vi "MEASURE_2dmapping.vi"() -> ()   [LabVIEW 2021]
uses:
  <vilib>/DAQmx/read.llb/DAQmx Read.vi
  <vilib>/DAQmx/read.llb/DAQmx Read (Counter U32 1Chan 1Samp).vi
  <vilib>/Analysis/baseanly.llb/Mean (DBL).vi
  <vilib>/DAQmx/create/channels.llb/DAQmx Create Channel (CI-Count Edges).vi
  <instrlib>/Keithley 24XX/Public/Data/Read (Multiple Points).vi
  <vilib>/DAQmx/miscellaneous.llb/DAQmx Fill In Error Info.vi
  <vilib>/Utility/file.llb/Write To Spreadsheet File (DBL).vi
  <instrlib>/Stanford Research 830/Stanford Research 830.lvlib
  <instrlib>/Keithley 2450/Keithley 2450.lvlib
  <resource>/objmgr/daqmx.rc
  <instrlib>/Keithley 24XX/Keithley 24XX.lvlib
  <vilib>/Analysis/NI_AALBase.lvlib
panel:
  out "XY Graph 4":cluster{dbl[], dbl[]}(graph)
  out "XY Graph 3":cluster{dbl[], dbl[]}(graph)
  out "top gate leaking":dbl
  out "top gate voltage":dbl format="%#_13g"
  in  "Compliance  Level (1uA)":dbl=1e-06
  in  "Source Mode  (0: Voltage)":u16(ring) items=["Voltage", "Current"]
  in  "Serial Configuration":T1={"Baud Rate"=9600, "Parity"=0, "Data Bits"=8, "Stop Bits"=10, "Flow Control"=0} {"Flow Control" items=["None", "XON/XOFF", "RTS/CTS", "XON/XOFF & RTS/CTS", "DTR/DSR", "XON/XOFF & DTR/DSR"]; "Stop Bits" items=["1.0"=10, "1.5"=15, "2.0"=20]; "Data Bits" items=["7"=7, "8"=8]; "Parity" items=["None", "Odd", "Even", "Mark", "Space"]; "Baud Rate" items=["300"=300, "600"=600, "1200"=1200, "2400"=2400, "4800"=4800, "9600"=9600, "19200"=19200]}
  in  "top gate address":refnum<visa-resource-name>="GPIB0::24::INSTR"
  in  "top gate thickness":dbl
  in  "bottom gate thickness":dbl
  in  "pure field (T)/pure doping (F)":bool
  in  "Clear Plot 2":bool
  out "XY Graph 2":cluster{dbl[], dbl[]}(graph)
  in  "accumulation":i32=100
  out "Waveform Chart 3":dbl[](graph)
  out "Numeric":dbl
  in  "Counter Channel":tag="/Dev1/PFI0"
  in  "error in":errorcluster
  out "loop run":i32
  in  "loop #":i32
  in  "Save data or not":bool=TRUE
  in  "path (folder + filename)":string="D:\\Kedar\\MoS2\\jw7_DJ_bulk_111213\\VvsHtr\\VvsHtr_300K"
  in  "Clear Plot":bool
  out "LOCKIN Measurement":dbl
  in  "Parameter (1: X)":u16(ring)=1 items=["X"=1, "Y"=2, "R"=3, "Theta"=4, "Channel 1"=5, "Channel 2"=6, "Aux In 1"=7, "Aux In 2"=8, "Aux In 3"=9, "Aux In 4"=10]
  out "back gate voltage":dbl format="%#_13g"
  out "back gate leaking":string="defbuffer1"
  in  "GATE STEP(mv)":i32
  in  "GATE Low Value (default 0)":dbl=1.0
  in  "GATE High Value":dbl=1.0
  in  "Function (0: Volts) 2":u16(ring) items=["Volts", "Current", "Resistance"]
  in  "Source Compaliance":dbl=1e-06
  in  "topgate address":refnum<visa-resource-name>="GPIB0::24::INSTR"
  in  "SD stabilization(S) 2":dbl format="%#_13g"
  in  "Sine Output Amplitude (1 V) 2":dbl=1.0
  in  "GATE / SD stablization 3":dbl format="%#_13g"
  in  "frequency":dbl format="%#_13g"
  in  "Input Connection (0: Single-Ended Voltage)":u16(ring) items=["Single-Ended Voltage", "Differential Voltage", "1 MOhm Current Gain", "100 MOhm Current Gain"]
  in  "LOCKIN address":refnum<visa-resource-name>="GPIB0::24::INSTR"
  # "Gate2450(back) Setting"
  # "Lock-in"
  # "Gate2401(top) Setting"
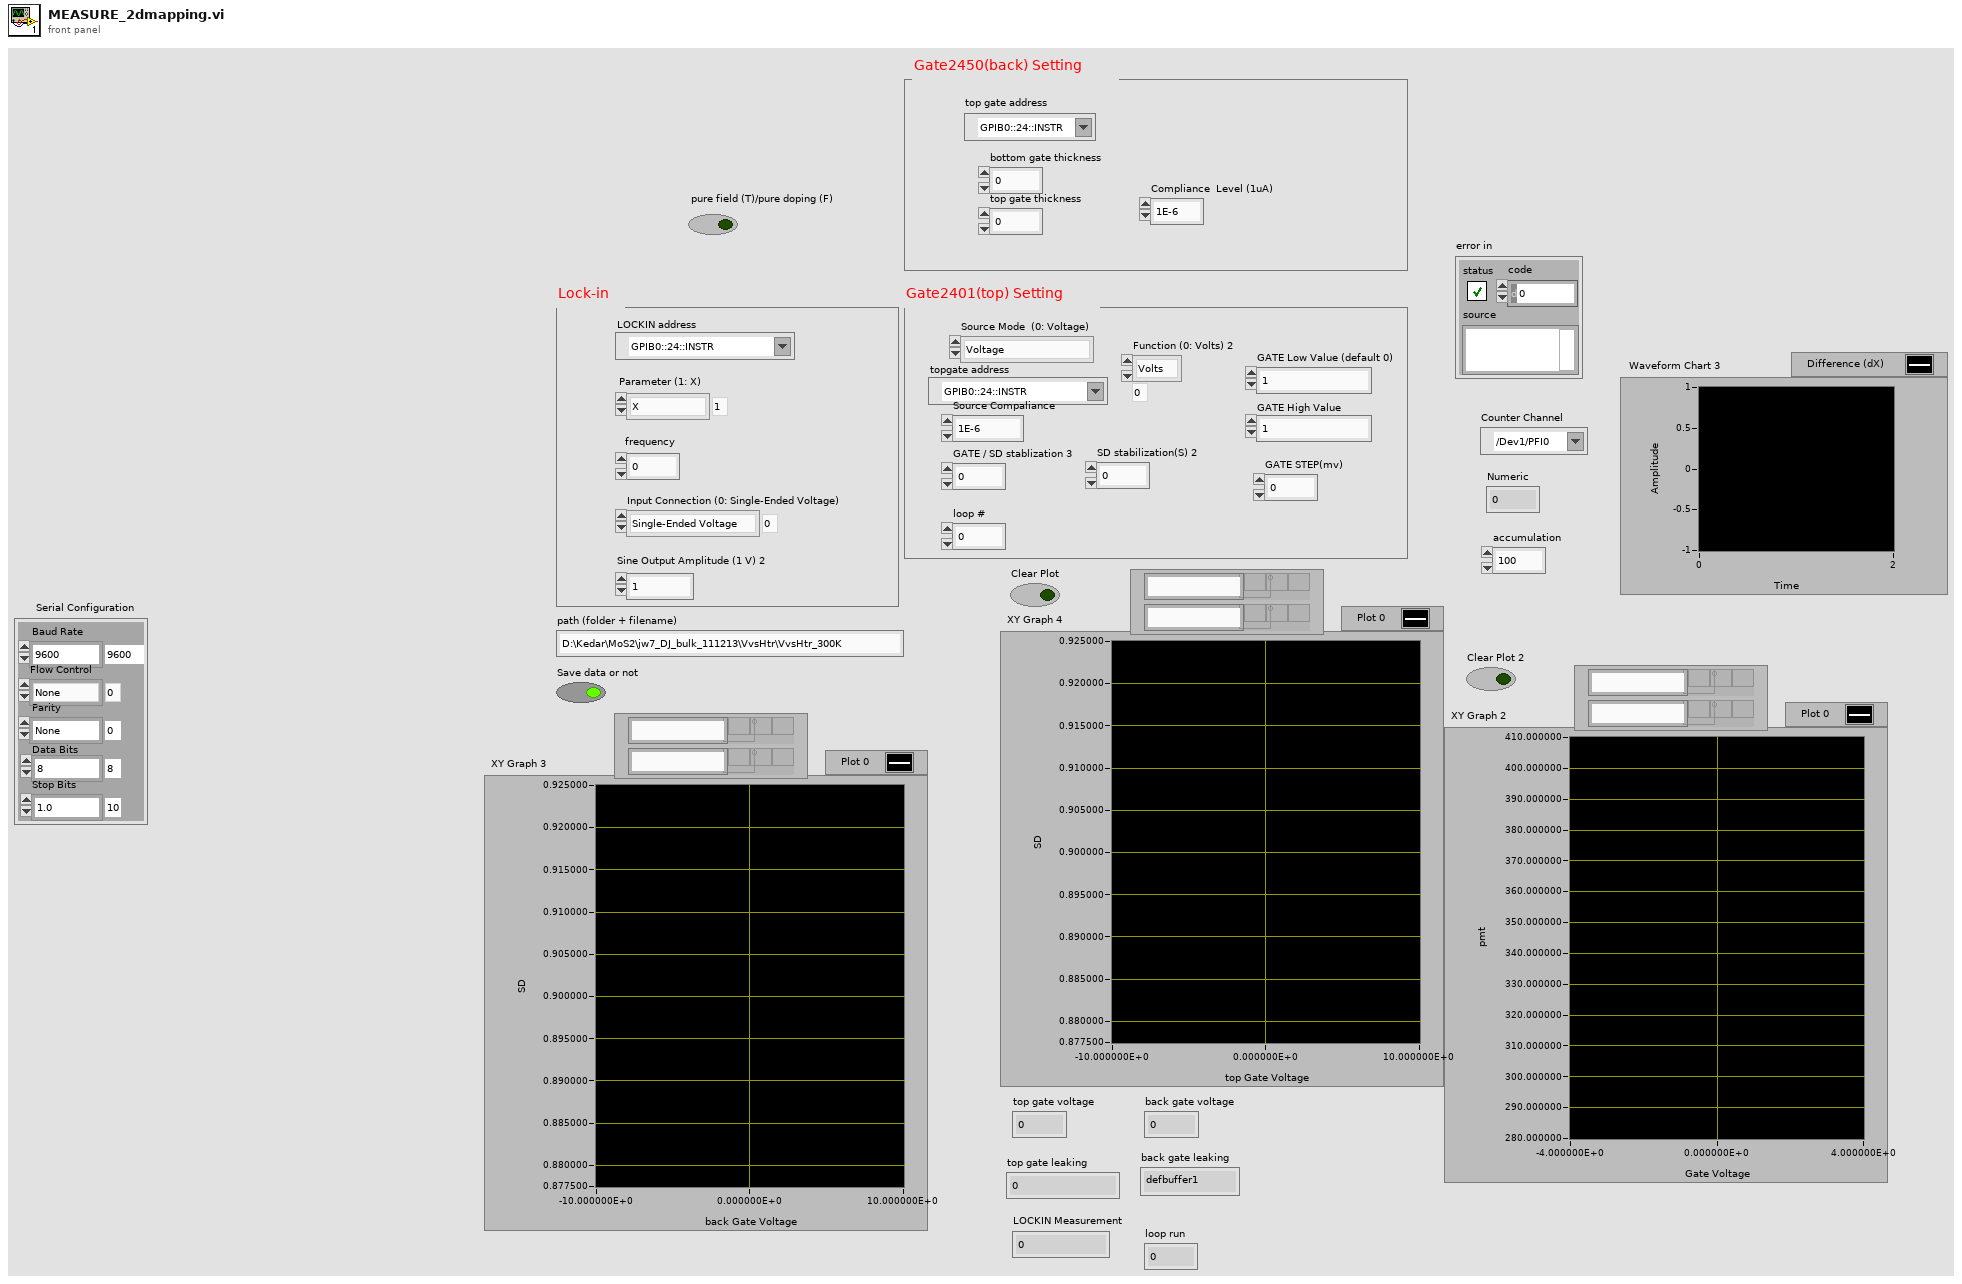
[diagram p1: front panel]
types:
  T1 = cluster{"Baud Rate":u32, "Parity":u16, "Data Bits":u16, "Stop Bits":u16, "Flow Control":u16}
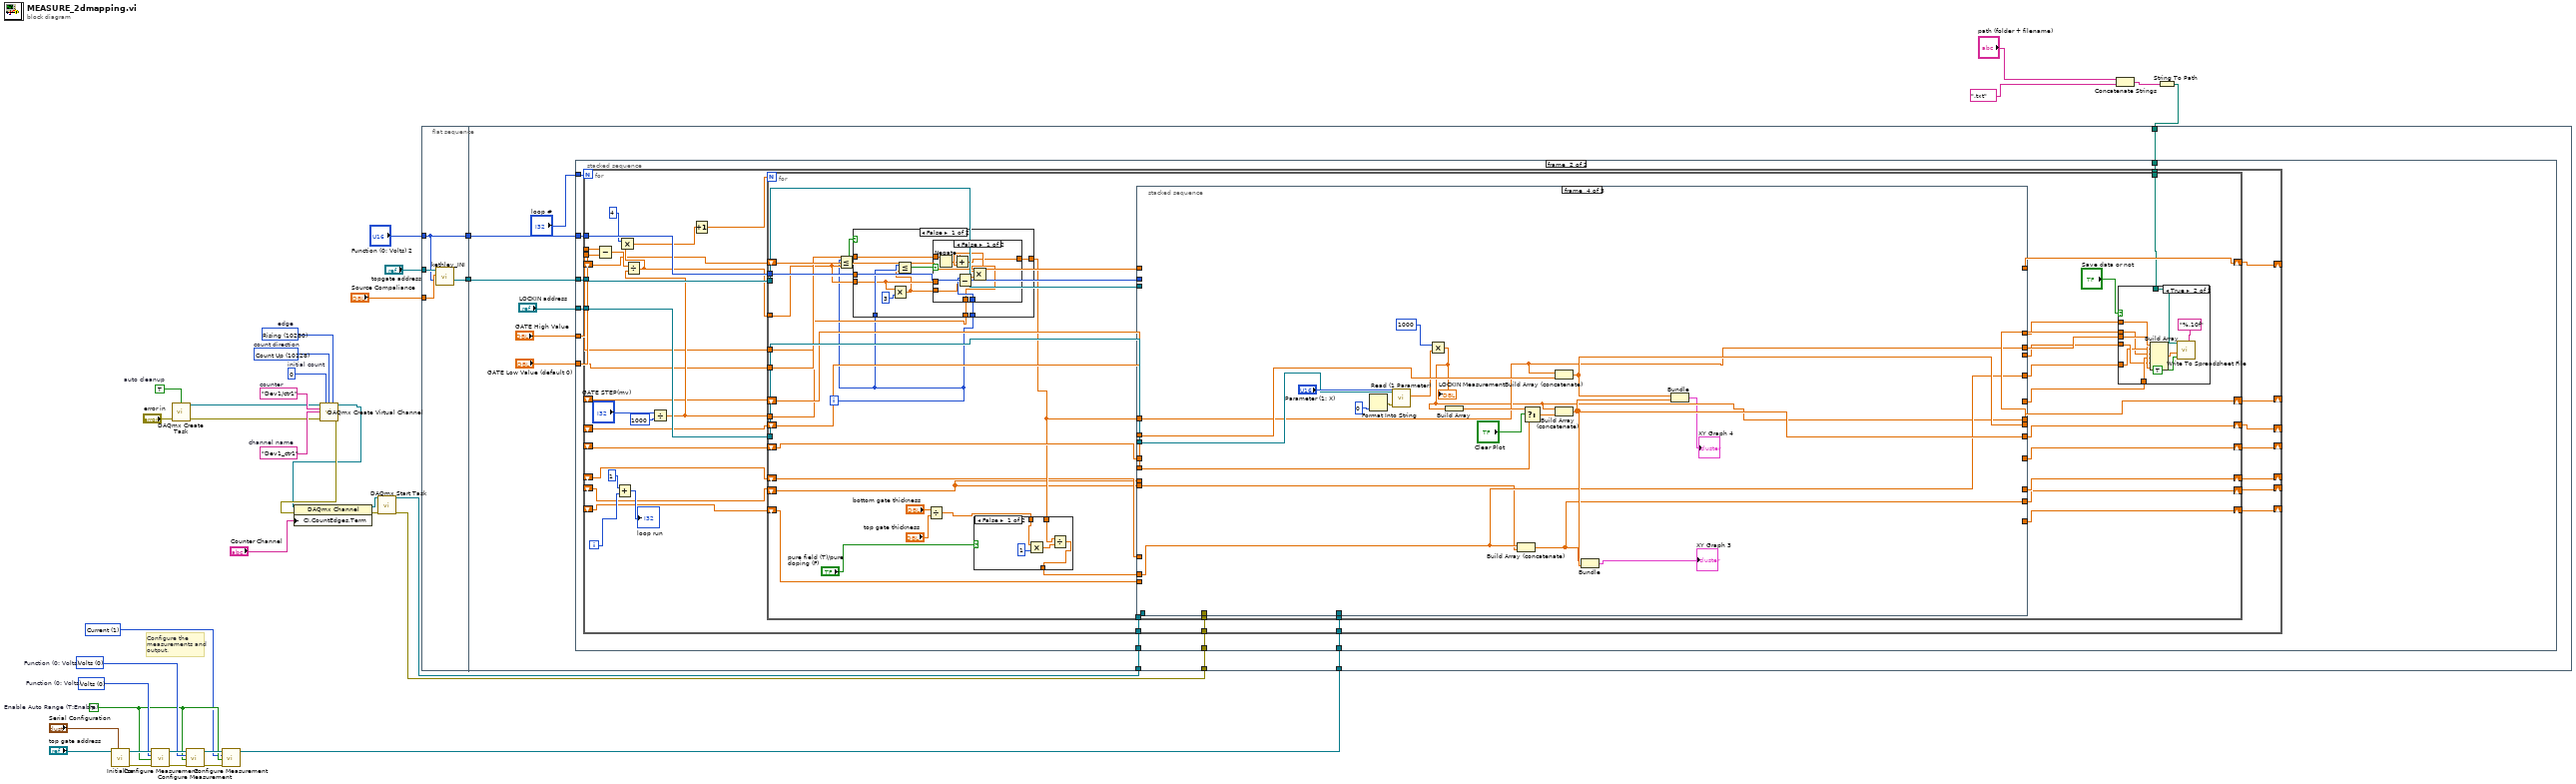
[diagram p0: block diagram]
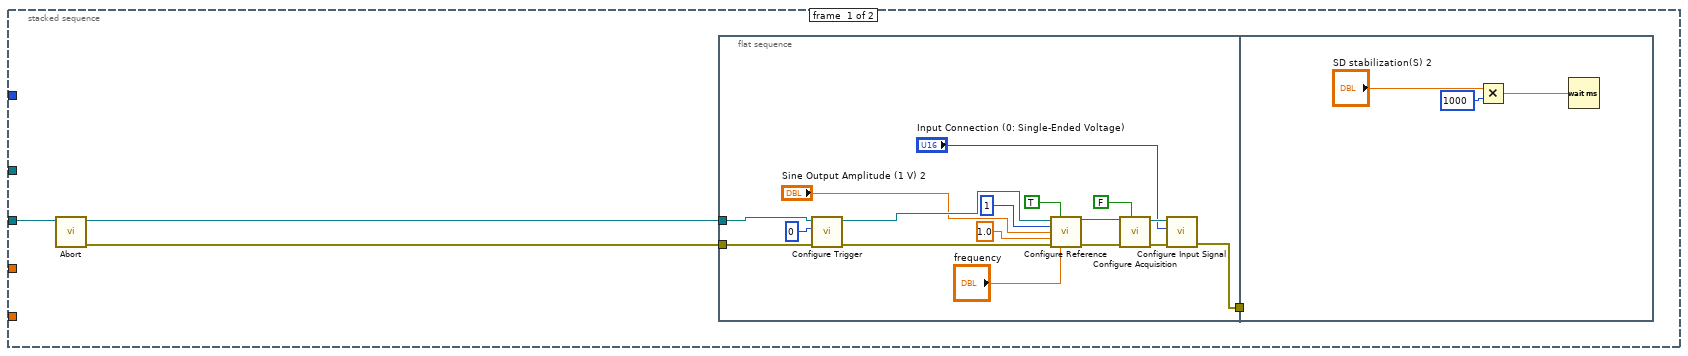
[diagram p2: hidden frame]
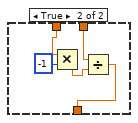
[diagram p3: hidden frame]
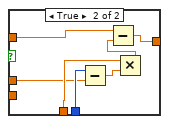
[diagram p5: hidden frame]
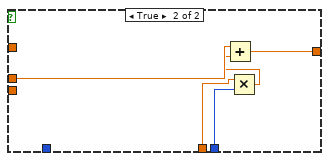
[diagram p6: hidden frame]
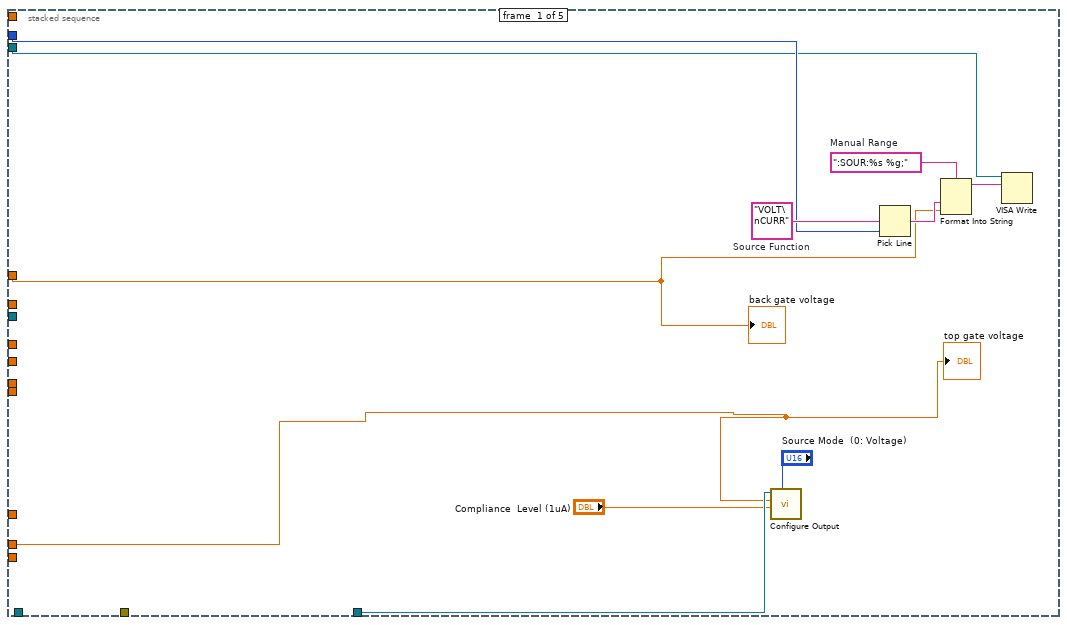
[diagram p7: hidden frame]
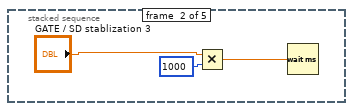
[diagram p8: hidden frame]
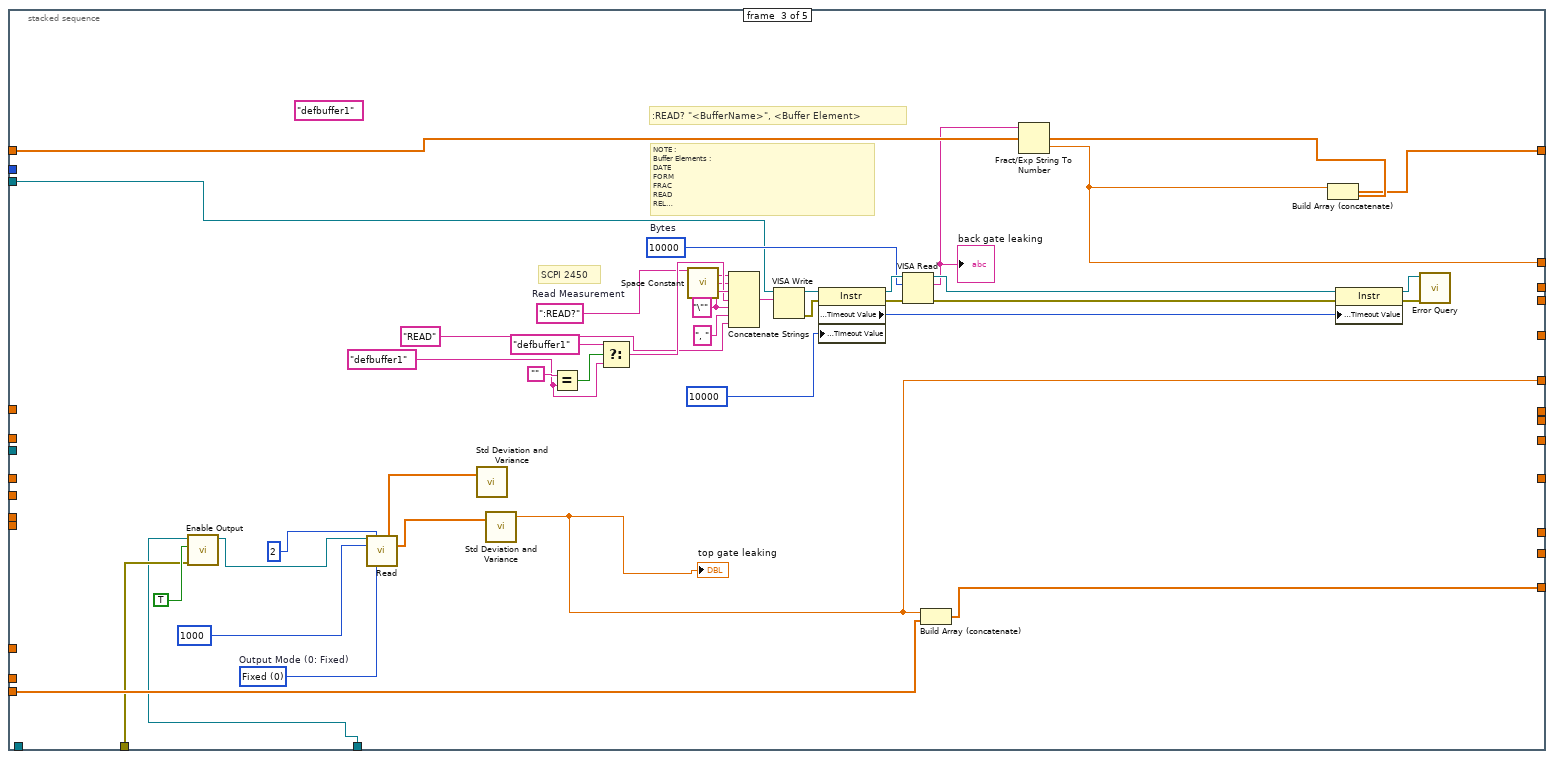
[diagram p9: hidden frame]
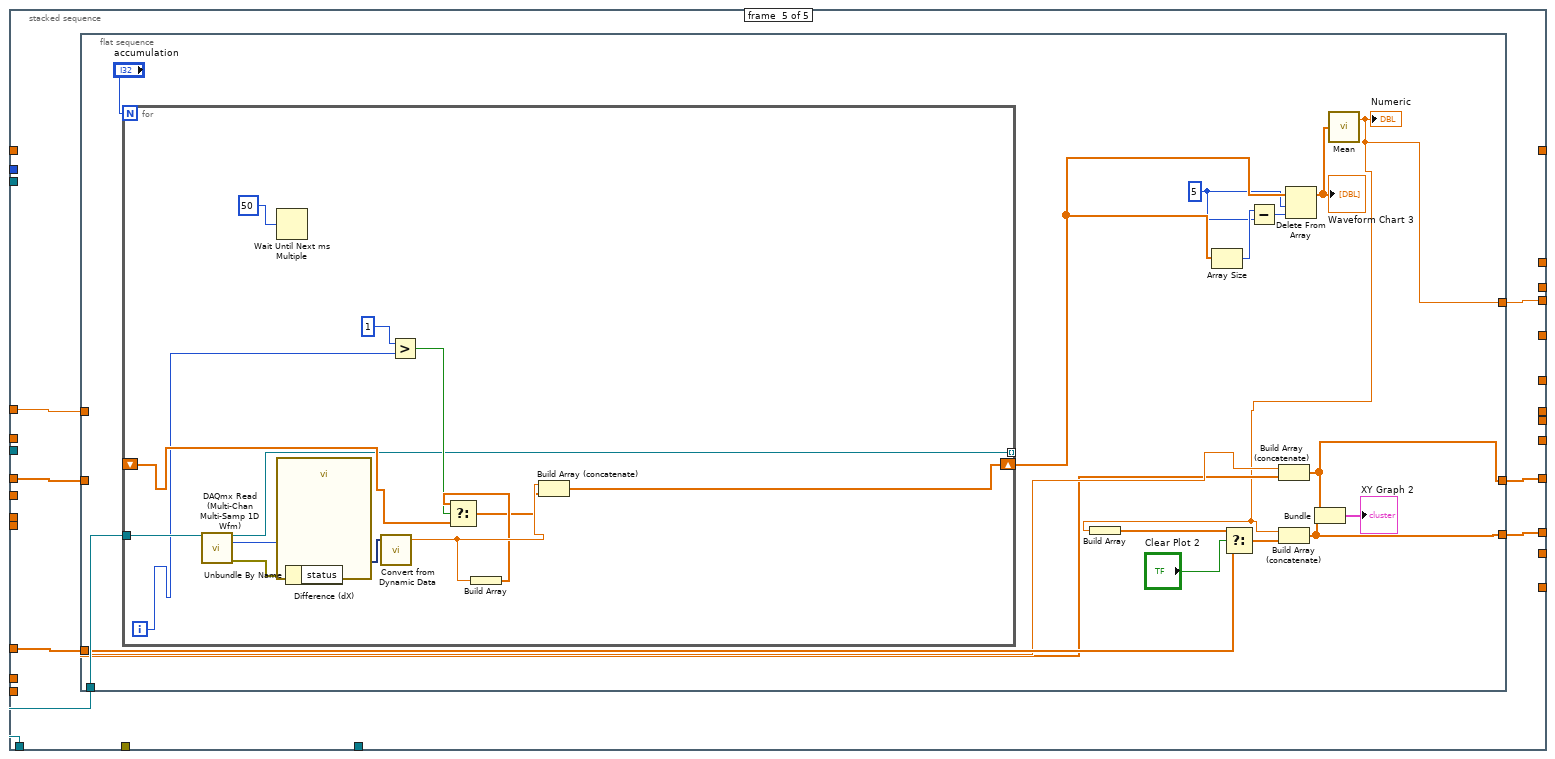
[diagram p10: hidden frame]
diagram:
  w3 = u16 1 items=["Volts", "Current", "Resistance"] ("Function (0: Volts)")
  w4 = TRUE  # Enable Auto Range (T:Enable)
  w7 = u16 0 items=["Volts", "Current", "Resistance"]  # Function (0: Volts)
  w8 = u16 0 items=["Volts", "Current", "Resistance"]  # Function (0: Volts)
  w27 = 10280 items=["Rising"=10280, "Falling"=10171]  # edge
  w26 = 10128 items=["Count Up"=10128, "Count Down"=10124, "Externally Controlled"=10326]  # count direction
  w25 = u32 0  # initial count
  w24 = "Dev1_ctr1"  # channel name
  w23 = "Dev1/ctr1"  # counter
  w21 = TRUE  # auto cleanup
  # "Configure the measurements and output."
  n1 = call <instrlib>:"Initialize.vi"("Serial Configuration"="Serial Configuration", "VISA resource name"="top gate address") -> ("error out"=w13:errorcluster, "VISA resource name out"=w14:refnum<visa-resource-name>)  [unwired: 8 in]
  n2 = call <instrlib>:"Configure Measurement.vi"("error in (no error)"=w13, "Enable Auto Range (T:Enable)"=w4, "Function (0: Volts)"=w8, "VISA resource name"=w14) -> ("error out"=w12:errorcluster, "VISA resource name out"=w11:refnum<visa-resource-name>)  [unwired: 6 in]
  n3 = call <vilib>:"DAQmx Create Task.vi"("auto cleanup"=w21, "error in"="error in") -> ("task out"=w22:refnum<k21>, "error out"=w20:errorcluster)  [unwired: 12 in]
  n4 = call <instrlib>:"Configure Measurement.vi"("error in (no error)"=w12, "Enable Auto Range (T:Enable)"=w4, "Function (0: Volts)"=w7, "VISA resource name"=w11) -> ("error out"=w5:errorcluster, "VISA resource name out"=w6:refnum<visa-resource-name>)  [unwired: 6 in]
  n5 = call <instrlib>:"Configure Measurement.vi"("error in (no error)"=w5, "Enable Auto Range (T:Enable)"=w4, "Function (0: Volts)"=w3, "VISA resource name"=w6) -> ("VISA resource name out"=w2:refnum<visa-resource-name>)  [unwired: 6 in, 1 out]
  n6 = call-poly <vilib>:"DAQmx Create Virtual Channel.vi"("task in"=w22, "initial count"=w25, "count direction"=w26, "edge"=w27, "counter"=w23, "name to assign"=w24, "error in"=w20) -> ("task out"=w28:refnum<k21>, "error out"=w29:errorcluster)  [unwired: 7 in]
  n7 = property class="DAQmx Channel"(reference=w28, error in=w29, "CI.CountEdges.Term"="Counter Channel") -> (reference out=w16:refnum<k21>, error out=w17:errorcluster)
  n8 = call <vilib>:"DAQmx Start Task.vi"("task/channels in"=w16, "error in"=w17) -> ("task out"=w15:refnum<k21>, "error out"=w1:errorcluster)  [unwired: 12 in]
  n9 = flat-sequence {
    tunnel: "topgate address" -> [w42]
    tunnel: "Source Compaliance" -> [w41]
    tunnel: "Function (0: Volts) 2" -> [w39]
    tunnel: [w40] -> w35
    tunnel: [w39] -> w34
    tunnel: w35 -> [w51]
    tunnel: w34 -> [w50]
    tunnel: w30 -> [w47]
    tunnel: w15 -> [w45]
    tunnel: w2 -> [w44]
    tunnel: w1 -> [w43]
    frame #0 {
      n10 = call "kethley_INI.vi"("Function (0: Volts) in"=w39, "Source Compaliance"=w41, "VISA Refnum in"=w42) -> ("VISA resource name out"=w40:refnum<visa-resource-name>)  [unwired: 8 in]
    }
    frame #1 {
      n11 = stacked-sequence {
        tunnel: "LOCKIN address" -> [w55 w84]
        tunnel: w51 -> [_ w85]
        tunnel: w50 -> [_ w86]
        tunnel: "GATE High Value" -> [_ w82]
        tunnel: "GATE Low Value (default 0)" -> [_ w83]
        tunnel: w47 -> [_ w81]
        tunnel: "loop #" -> [_ w80]
        tunnel: w45 -> [_ w79]
        tunnel: w44 -> [_ w78]
        tunnel: w43 -> [_ w77]
        frame #0 {
          n12 = call <instrlib>:"Abort.vi"("VISA resource name"=w55) -> ("error out"=w53:errorcluster, "VISA resource name out"=w54:refnum<visa-resource-name>)  [unwired: 9 in]
          n13 = flat-sequence {
            tunnel: w54 -> [w73]
            tunnel: [w58] -> w56
            tunnel: w53 -> [w57]
            tunnel: w56 -> [_]
            frame #0 {
              n14 = call <instrlib>:"Configure Trigger.vi"("error in (no error)"=w57, "Trigger Source (0: Internal)"=0, "VISA resource name"=w73) -> ("error out"=w67:errorcluster, "VISA resource name out"=w68:refnum<visa-resource-name>)  [unwired: 7 in]
              n15 = call <instrlib>:"Configure Reference.vi"("VISA resource name"=w68, "Auto Phase (T: Enabled)"=TRUE, "Reference Source (1: Internal)"=1, "Sine Output Amplitude (1 V)"="Sine Output Amplitude (1 V) 2", "Detection Harmonic Number (1)"=1.0 ("output voltage 2"), "error in (no error)"=w67, "Internal Reference Frequency (1000 Hz)"="frequency") -> ("VISA resource name out"=w65:refnum<visa-resource-name>, "error out"=w60:errorcluster)  [unwired: 7 in]
              n16 = call <instrlib>:"Configure Acquisition.vi"("Continuous Storage (T: Enable)"=FALSE, "error in (no error)"=w60, "VISA resource name"=w65) -> ("error out"=w59:errorcluster, "VISA resource name out"=w63:refnum<visa-resource-name>)  [unwired: 7 in]
              n17 = call <instrlib>:"Configure Input Signal.vi"("error in (no error)"=w59, "Input Connection (0: Single-Ended Voltage)"="Input Connection (0: Single-Ended Voltage)", "VISA resource name"=w63) -> ("error out"=w58:errorcluster)  [unwired: 7 in, 1 out]
            }
            frame #1 {
              n18 = Multiply(x="SD stabilization(S) 2", y=1000) -> (x*y=w76:dbl)
              n19 = Wait (ms)(milliseconds to wait=w76) -> ()  [unwired: 1 out]
            }
          }
        }
        frame #1 {
          n20 = for {
            N: w80 -> [_]
            tunnel: w86 -> [w120]
            tunnel: w85 -> [w119]
            tunnel: w84 -> [w118]
            tunnel: w83 -> [w112]
            tunnel: w82 -> [w111]
            tunnel: w81 -> [w110]
            shift-right: [w106] -> _
            shift-left: _ -> [w105]
            shift-right: [w104] -> _
            shift-left: _ -> [w102]
            shift-right: [w103] -> _
            shift-left: _ -> [w101]
            tunnel: w79 -> [w97]
            shift-right: [w96] -> _
            shift-left: _ -> [w95]
            shift-right: [w94] -> _
            shift-left: _ -> [w93]
            shift-right: [w92] -> _
            shift-left: _ -> [w91]
            shift-right: [w90] -> _
            shift-left: _ -> [w89]
            tunnel: w78 -> [w88]
            tunnel: w77 -> [w87]
            i -> [w99]
            n21 = Subtract(x=w111, y=w112) -> (x-y=w114:dbl)
            n22 = Add(x=1, y=w99) -> (x+y=→"loop run":i32)
            n23 = Divide(x="GATE STEP(mv)", y=1000) -> (x/y=w113:dbl)
            n24 = Divide(x=w114, y=w113) -> (x/y=w109:dbl)
            n25 = Multiply(x=4, y=w109) -> (x*y=w108:dbl)
            n26 = Increment(x=w108) -> (x+1=w107:dbl)
            n27 = for {
              N: w107 -> [_]
              tunnel: w120 -> [w160]
              tunnel: w119 -> [w159]
              tunnel: w118 -> [w158]
              tunnel: w113 -> [w149]
              shift-right: [w157] -> w106
              shift-left: w105 -> [w156]
              shift-right: [w153] -> w103
              shift-left: w101 -> [w155]
              shift-right: [w152] -> w104
              shift-left: w102 -> [w154]
              tunnel: w109 -> [w147]
              tunnel: w112 -> [w150]
              tunnel: w111 -> [w148]
              tunnel: w110 -> [w142]
              tunnel: w97 -> [w140]
              shift-right: [w139] -> w96
              shift-left: w95 -> [w124]
              shift-right: [w138] -> w94
              shift-left: w93 -> [w137]
              shift-right: [w135] -> w92
              shift-left: w91 -> [w125]
              shift-right: [w134] -> w90
              shift-left: w89 -> [w123]
              tunnel: w88 -> [w132]
              tunnel: w87 -> [w122]
              i -> [w146]
              n28 = Less Or Equal?(x=w146, y=w147) -> (x <= y?=w151:bool)
              n29 = case shown="False" w151 {
                tunnel: w150 -> [_ w209]
                tunnel: w146 -> [w189 w208]
                tunnel: w149 -> [w188 w207]
                tunnel: [w186 w205] -> w127
                tunnel: w148 -> [w187 _]
                tunnel: w147 -> [w182 _]
                tunnel: w146 -> [w185 _]
                frame False {
                  n30 = Multiply(x=w182, y=3) -> (x*y=w181:dbl)
                  n31 = Less Or Equal?(x=w185, y=w181) -> (x <= y?=w183:bool)
                  n32 = case shown="False" w183 {
                    tunnel: w189 -> [w197 w204]
                    tunnel: w188 -> [w195 w202]
                    tunnel: w187 -> [w191 w200]
                    tunnel: [w193 w199] -> w186
                    tunnel: w182 -> [_ w198]
                    tunnel: w181 -> [w190 _]
                    frame False {
                      n33 = Negate(x=w191) -> (-x=w192:dbl)
                      n34 = Subtract(x=w197, y=w190) -> (x-y=w196:dbl)
                      n35 = Multiply(x=w195, y=w196) -> (x*y=w194:dbl)
                      n36 = Add(x=w192, y=w194) -> (x+y=w193:dbl)
                    }
                    frame True {
                      n37 = Subtract(x=w204, y=w198) -> (x-y=w203:dbl)
                      n38 = Multiply(x=w202, y=w203) -> (x*y=w201:dbl)
                      n39 = Subtract(x=w200, y=w201) -> (x-y=w199:dbl)
                    }
                  }
                }
                frame True {
                  n40 = Multiply(x=w207, y=w208) -> (x*y=w206:dbl)
                  n41 = Add(x=w209, y=w206) -> (x+y=w205:dbl)
                }
              }
              n42 = Divide(x="bottom gate thickness", y="top gate thickness") -> (x/y=w131:dbl)
              n43 = case shown="False" "pure field (T)/pure doping (F)" {
                tunnel: w131 -> [w164 w170]
                tunnel: [w161 w168] -> w126
                tunnel: w127 -> [w162 w167]
                frame False {
                  n44 = Multiply(x=w164, y=1) -> (x*y=w163:dbl)
                  n45 = Divide(x=w162, y=w163) -> (x/y=w161:dbl)
                }
                frame True {
                  n46 = Multiply(x=w170, y=-1) -> (x*y=w166:dbl)
                  n47 = Divide(x=w167, y=w166) -> (x/y=w168:dbl)
                }
              }
              n48 = stacked-sequence {
                tunnel: w160 -> [w216 _ _ _ _]
                tunnel: w159 -> [w215 _ w240 _ _]
                tunnel: w158 -> [_ _ _ w274 _]
                tunnel: w127 -> [w214 _ _ w273 w285]
                tunnel: [_ _ w238 _ _] -> w157
                tunnel: w156 -> [_ _ w239 _ _]
                tunnel: w155 -> [_ _ _ w277 _]
                tunnel: w154 -> [_ _ _ w275 _]
                tunnel: [_ _ _ w270 _] -> w153
                tunnel: [_ _ _ w276 _] -> w152
                tunnel: [_ _ _ w264 _] -> w145
                tunnel: [_ _ _ w273 _] -> w144
                tunnel: [_ _ w236 _ _] -> w143
                tunnel: w140 -> [_ _ _ _ w289]
                tunnel: [_ _ _ _ w288] -> w139
                tunnel: w124 -> [_ _ _ _ w287]
                tunnel: [_ _ _ _ w286] -> w138
                tunnel: w137 -> [_ _ _ _ w284]
                tunnel: [_ _ _ _ w283] -> w136
                tunnel: [_ _ w230 _ _] -> w135
                tunnel: [_ _ _ w269 _] -> w134
                tunnel: w123 -> [_ _ _ _ _]
                tunnel: [_ _ _ w268 _] -> w133
                tunnel: [_ _ w229 _ _] -> w121
                tunnel: w132 -> [w212 _ w225 _ _]
                tunnel: w126 -> [w210 _ _ w268 _]
                tunnel: w125 -> [_ _ w228 _ _]
                tunnel: w123 -> [_ _ _ w267 _]
                tunnel: w122 -> [_ _ w226 _ _]
                frame #0 {
                  w218 = "VOLT\nCURR"  # Source Function
                  w219 = ":SOUR:%s %g;"  # Manual Range
                  n49 = call <instrlib>:"Configure Output.vi"("Source Mode  (0: Voltage)"="Source Mode  (0: Voltage)", "Compliance  Level (0.1)"="Compliance  Level (1uA)", "Output Level (0)"=w210, "VISA resource name"=w212) -> ()  [unwired: 6 in, 2 out]
                  n50 = Pick Line(multi-line string=w218, line index=w216) -> (output string=w217:string)  [unwired: 1 out]
                  n51 = Format Into String(format string=w219, w217, w214) -> (resulting string=w220:string)  [unwired: 2 in, 1 out]
                  n52 = VISA Write(VISA resource name=w215, write buffer=w220) -> ()  [unwired: 1 in, 3 out]
                  "back gate voltage" <- w214
                  "top gate voltage" <- w210
                }
                frame #1 {
                  n53 = Multiply(x="GATE / SD stablization 3", y=1000) -> (x*y=w223:dbl)
                  n54 = Wait (ms)(milliseconds to wait=w223) -> ()  [unwired: 1 out]
                }
                frame #2 {
                  w233 = u16 0 items=["Fixed", "Sweep", "List"]  # Output Mode (0: Fixed)
                  w251 = "defbuffer1" ("Buffer Name (defbuffer1) 2")
                  (unwired) "defbuffer1" ("t")
                  w249 = "\""
                  w246 = ":READ?"  # Read Measurement
                  w255 = u32 10000  # Bytes
                  # "NOTE :\nBuffer Elements :\nDATE\nFORM\nFRAC\nREAD\nREL\nSEC\nSOUR\nSOURFORM\nSOURSTAT\nSOURUNIT\nSTAT\nTIME\nTsT\nUNIT"
                  # ":READ? \"<BufferName>\", <Buffer Element>"
                  # "SCPI 2450"
                  n55 = call <instrlib>:"Enable Output.vi"("error in (no error)"=w226, "Enable Output (T: Enable)"=TRUE, "VISA resource name"=w225) -> ("VISA resource name out"=w224:refnum<visa-resource-name>)  [unwired: 7 in, 1 out]
                  n56 = call-poly <instrlib>:"Read.vi"("VISA resource name"=w224, "Sample Count (1)"=u32 2 ("Number of Samples"), "Timeout (10000 ms)"=1000, "Output Mode (0: Fixed)"=w233) -> ("Voltage"=w231:sgl[], "Current"=w232:sgl[])  [unwired: 5 in, 5 out]
                  n57 = call <vilib>:"Std Deviation and Variance.vi"("X"=w231) -> ()  [unwired: 1 in, 3 out]
                  n58 = call <vilib>:"Std Deviation and Variance.vi"("X"=w232) -> ("mean"=w229:dbl)  [unwired: 1 in, 2 out]
                  "top gate leaking" <- w229
                  n59 = Equal?(x="", y=w251) -> (x = y?=w252:bool)
                  n60 = Select(t="defbuffer1", s=w252, f=w251) -> (s? t:f=w248:string)
                  n61 = call <vilib>:"Space Constant.vi"() -> ("String"=w247:string)
                  n62 = Concatenate Strings(w246, w247, w249, w248, w249, ", " ("string"), "READ" ("Buffer Elements 2")) -> (w262:string)
                  n63 = VISA Write(VISA resource name=w240, write buffer=w262) -> (VISA resource name out=w254:refnum<visa-resource-name>, error out=w261:errorcluster)  [unwired: 1 in, 1 out]
                  n64 = property class="Instr"(reference=w254, error in=w261, "General Settings:Timeout Value"=10000 ("Timeout (10000 ms) 2")) -> (reference out=w260:refnum<visa-resource-name>, error out=w259:errorcluster, "General Settings:Timeout Value"=w256:u32)
                  n65 = VISA Read(VISA resource name=w260, byte count=w255, error in (no error)=w259) -> (VISA resource name out=w258:refnum<visa-resource-name>, read buffer=w237:string, error out=w257:errorcluster)  [unwired: 1 out]
                  "back gate leaking" <- w237
                  n66 = Build Array (concatenate)(w229, w228) -> (w230:dbl[])
                  n67 = Fract/Exp String To Number(string=w237) -> (number=w236:dbl)  [unwired: 3 in, 1 out]
                  n68 = Build Array (concatenate)(w236, w239) -> (w238:dbl[])
                  n69 = property class="Instr"(reference=w258, error in=w257, "General Settings:Timeout Value"=w256) -> (reference out=w244:refnum<visa-resource-name>, error out=w243:errorcluster)
                  n70 = call <instrlib>:"Error Query.vi"("error in (no error)"=w243, "VISA resource name"=w244) -> ()  [unwired: 10 out]
                }
                frame #3 {
                  n71 = Format Into String(0) -> (error out=w282:errorcluster)  [unwired: 3 in, 1 out]
                  n72 = call <instrlib>:"Read (1 Parameter).vi"("error in (no error)"=w282, "Parameter (1: X)"="Parameter (1: X)", "VISA resource name"=w274) -> ("Measurement"=w265:dbl)  [unwired: 6 in, 2 out]
                  n73 = Multiply(x=1000, y=w265) -> (x*y=w264:dbl)
                  "LOCKIN Measurement" <- w264
                  n74 = Build Array(w264) -> (w280:dbl[])
                  n75 = Build Array (concatenate)(w268, w267) -> (w269:dbl[])
                  n76 = Select(t=w280, s="Clear Plot", f=w277) -> (s? t:f=w272:dbl[])
                  n77 = Build Array (concatenate)(w273, w275) -> (w276:dbl[])
                  n78 = Build Array (concatenate)(w264, w272) -> (w270:dbl[])
                  n79 = Bundle(w269, w270) -> (→"XY Graph 3":cluster{dbl[], dbl[]})  [unwired: 1 in]
                  n80 = Bundle(w276, w270) -> (→"XY Graph 4":cluster{dbl[], dbl[]})  [unwired: 1 in]
                }
                frame #4 {
                  n81 = flat-sequence {
                    tunnel: w289 -> [w301]
                    tunnel: [w294] -> w288
                    tunnel: w287 -> [w295]
                    tunnel: [w293] -> w286
                    tunnel: w285 -> [w292]
                    tunnel: w284 -> [w291]
                    tunnel: [w290] -> w283
                    frame #0 {
                      w303 = 5
                      n82 = for {
                        N: "accumulation" -> [_]
                        tunnel: w301 -> [w311]
                        shift-right: [w310] -> w305
                        shift-left: _ -> [w309]
                        tunnel: [w307] -> _ mode=indexing
                        i -> [w308]
                        n83 = call-poly "DAQmx Read (Multi-Chan Multi-Samp 1D Wfm).vi"("task/channels in"=w311) -> ("task out"=w307:refnum<k21>, "data"=w317:u32, "error out"=w318:errorcluster)  [unwired: 12 in]
                        n84 = Wait Until Next ms Multiple(millisecond multiple=50) -> ()  [unwired: 1 out]
                        n85 = call "Difference (dX)"("Signals"=w317) -> ("Result"=w320:dynamicdata)  [unwired: 5 in, 1 out]
                        n86 = Unbundle By Name(w318) -> ()  [unwired: 1 out]
                        n87 = call "Convert from Dynamic Data"("Dynamic Data Type"=w320) -> ("Scalar"=w316:dbl)  [unwired: 3 in]
                        n88 = Greater?(x=1, y=w308) -> (0:w312:bool)
                        n89 = Build Array(w316) -> (w315:dbl[])
                        n90 = Select(t=w315, s=w312, f=w309) -> (s? t:f=w314:dbl[])
                        n91 = Build Array (concatenate)(w316, w314) -> (w310:dbl[])
                      }
                      n92 = Array Size(array=w305) -> (size(s)=w304:i32)
                      n93 = Subtract(x=w304, y=w303) -> (x-y=w302:i32)
                      n94 = Build Array (concatenate)(w292, w291) -> (w293:dbl[])
                      n95 = Delete From Array(array=w305, length=w303, index=w302) -> (array with subset deleted=w300:dbl[])  [unwired: 1 out]
                      "Waveform Chart 3" <- w300
                      n96 = call-poly <vilib>:"Mean.vi"("X"=w300) -> ("mean"=w290:dbl)  [unwired: 1 out]
                      "Numeric" <- w290
                      n97 = Build Array(w290) -> (w298:dbl[])
                      n98 = Select(t=w298, s="Clear Plot 2", f=w295) -> (s? t:f=w299:dbl[])
                      n99 = Build Array (concatenate)(w290, w299) -> (w294:dbl[])
                      n100 = Bundle(w293, w294) -> (→"XY Graph 2":cluster{dbl[], dbl[]})  [unwired: 1 in]
                    }
                  }
                }
              }
              n101 = case shown="True" "Save data or not" {
                tunnel: w145 -> [_ w171]
                tunnel: w144 -> [_ w180]
                tunnel: w143 -> [_ w179]
                tunnel: w142 -> [_ w177]
                tunnel: w136 -> [_ w173]
                tunnel: w133 -> [_ w172]
                tunnel: w121 -> [_ w174]
                frame False {
                }
                frame True {
                  n102 = Build Array(w180, w172, w171, w174, w173, w179) -> (w178:dbl[])
                  n103 = call-poly <vilib>:"Write To Spreadsheet File.vi"("format (%.3f)"="%.10f", "append to file? (new file:F)"=TRUE, "1D data"=w178, "file path (dialog if empty)"=w177) -> ()  [unwired: 4 in, 1 out]
                }
              }
            }
          }
        }
      }
    }
  }
  n104 = Concatenate Strings("path (folder + filename)", ".txt") -> (w31:string)
  n105 = String To Path(string=w31) -> (path=w30:path)
